vi "Startup_CheckFolders.vi"(8 "error in (no error)":errorcluster, 10 "Message Steps Ref In":refnum<vi>, 11 "MainVIPathIn":path) -> (0 "error out":errorcluster, 2 "Message Steps Ref Out":refnum<vi>, 3 "MainVIPathOut":path)   [LabVIEW 2016]
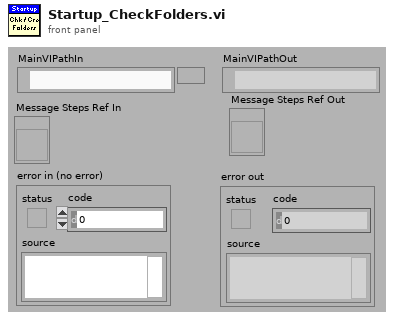
[diagram p1: front panel]
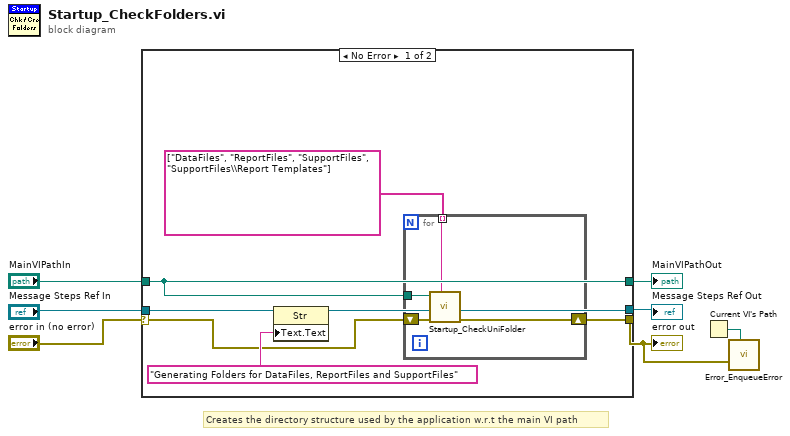
[diagram p0: block diagram]
diagram:
  # "Creates the directory structure used by the application w.r.t the main VI path"
  n1 = case shown="No Error" "error in (no error)" {
    selector: "error in (no error)" -> [w8 w21]
    tunnel: [w13 w21] -> w1
    tunnel: "MainVIPathIn" -> [w12 w20]
    tunnel: [w12 w20] -> w6
    tunnel: "Message Steps Ref In" -> [w11 w19]
    tunnel: [w10 w19] -> w3
    frame No Error {
      n2 = property class="Str"(reference=w11, "Text.Text"="Generating Folders for DataFiles, ReportFiles and SupportFiles") -> (reference out=w10:refnum<vi>)  [unwired: 1 in, 1 out]
      n3 = for {
        tunnel: string[] ["DataFiles", "ReportFiles", "SupportFiles", "SupportFiles\\Report Templates"] -> [w15] mode=indexing
        shift-right: [w16] -> w13
        shift-left: w8 -> [w17]
        tunnel: w12 -> [w18]
        n4 = call "Startup_CheckUniFolder.vi"("element"=w15, "error in"=w17, "path"=w18) -> ("error out"=w16:errorcluster)  [unwired: 8 out]
      }
    }
    frame Error {
    }
  }
  "error out" <- w1
  "MainVIPathOut" <- w6
  "Message Steps Ref Out" <- w3
  n5 = Current VI's Path() -> (path=w2:path)
  n6 = call "Error_EnqueueError.vi"("SourcePath"=w2, "Error in"=w1) -> ()  [unwired: 1 in, 9 out]
